vi "Send_Arm_Keithley.vi"(7 "Filename (.ini)":string="Config_Ver_1\\Keithley_params.ini", 8 "error in":errorcluster, 11 "Keithley VISA in":refnum<visa-resource-name>) -> (0 "error out":errorcluster, 2 "Trig Layer Params Out":T1, 3 "Keithley VISA out":refnum<visa-resource-name>)   [LabVIEW 2021]
uses:
  <instrlib>/Keithley 622x LV 2009/Configure/Trigger/Typedefs/KE622x -- Trig Layer Params.ctl
  <instrlib>/Keithley 622x LV 2009/Configure/Trigger/Low Level/Typedefs/KE622x -- Trig Source.ctl
  <instrlib>/Keithley 622x LV 2009/Configure/Trigger/Low Level/Typedefs/KE622x -- Trig Link Line.ctl
  <instrlib>/Keithley 622x LV 2009/Configure/Trigger/Low Level/Typedefs/KE622x -- Trig Output Mode.ctl
  <instrlib>/Keithley 622x LV 2009/Configure/Source/Typedefs/KE622x -- Sweep Type.ctl
  <instrlib>/Keithley 622x LV 2009/Keithley 622x.lvlib
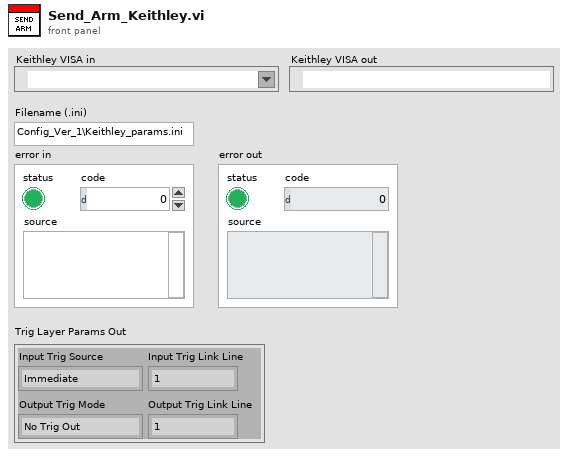
[diagram p1: front panel]
types:
  T1 = typedef "Keithley 622x.lvlib/KE622x -- Trig Layer Params.ctl" = cluster{"Input Trig Source":T2, "Input Trig Link Line":T3, "Output Trig Mode":T4, "Output Trig Link Line":T3}
  T2 = typedef "Keithley 622x.lvlib/KE622x -- Trig Source.ctl" = enum16{"Immediate", "Trigger Link"}
  T3 = typedef "Keithley 622x.lvlib/KE622x -- Trig Link Line.ctl" = enum16{"1", "2", "3", "4", "5", "6"}
  T4 = typedef "Keithley 622x.lvlib/KE622x -- Trig Output Mode.ctl" = enum16{"No Trig Out", "Source Turn On", "After Source Delay"}
  T5 = typedef "Keithley 622x.lvlib/KE622x -- Sweep Type.ctl" = enum16{"Linear", "Log", "List"}
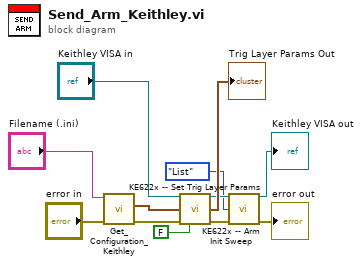
[diagram p0: block diagram]
diagram:
  n1 = call "Get_Configuration_Keithley.vi"("error in"="error in", "Filename (.ini)"="Filename (.ini)") -> ("error out"=w6:errorcluster, "Trig Layer Params In"=w10:T1)  [unwired: 5 in, 3 out]
  n2 = call <instrlib>:"KE622x -- Set Trig Layer Params.vi"("Resource In"="Keithley VISA in", "Trig Layer Params In"=w10, "error in (no error)"=w6, "Read Back Set Values? (T)"=FALSE) -> ("Resource Out (dupl)"=w5:refnum<visa-resource-name>, "Trig Layer Params Out"=→"Trig Layer Params Out":T1, "error out"=w4:errorcluster)  [unwired: 9 in]
  n3 = call <instrlib>:"KE622x -- Arm Init Sweep.vi"("Resource In"=w5, "Sweep Type"=KE622x_--_Sweep_Type."List", "error in (no error)"=w4) -> ("Resource Out (dupl)"=→"Keithley VISA out":refnum<visa-resource-name>, "error out"=→"error out":errorcluster)  [unwired: 11 in]
